vi "2d_Init.vi"(8 "error in (no error)":errorcluster, 11 "MagSpec_Bella in":refnum<class "MagSpec_Bella.lvclass">) -> (0 "error out":errorcluster, 3 "MagSpec_Bella out":refnum<class "MagSpec_Bella.lvclass">)   [LabVIEW 2020, in "MagSpec_Bella.lvclass"]
uses:
  MagSpec_Bella.lvclass
  MagSpec_Bella.lvclass/MagSpec_Bella.ctl
  2D.ctl
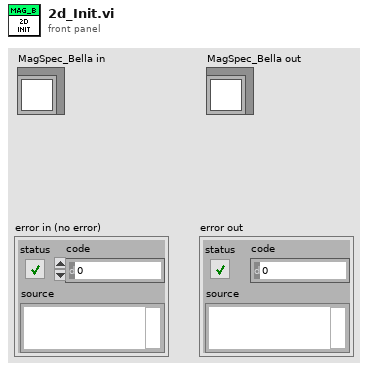
[diagram p1: front panel]
types:
  T1 = typedef "CameraSettings_File.ctl" = cluster{"FOV [mm]":dbl, "Left edge [mm]":dbl, "ROI Y offset":dbl, "ROI height":dbl, "ROI X offset":dbl, "ROI width":dbl, "Y center pixel":dbl, "Y Start":dbl, "Y End":dbl, "X Start":dbl, "X End":dbl, "rot [deg]":dbl}
  T2 = typedef "Calibration_Pixel_based.ctl" = cluster{"y1(pixel)":dbl[], "y2(pixel)":dbl[], "dp/B [MeV/C/B] (pixel)":dbl[], "energyDependence Input(pixel)":dbl[], "bending angle [deg](pixel)":dbl[], "total path(pixel)":dbl[], "pixel angle (y)(pixel)":dbl[], "energy dependence (pixel)":dbl[], "charge compensation (pixel)":dbl[], "Momentum [MeV/C](pixel)":dbl[], "angular compensation(pixel)":dbl[]}
  T3 = typedef "2D.ctl" = cluster{"dp":dbl[][], "chargeCompensation":dbl[][], "angle":dbl[][], "Momentum":dbl[][]}
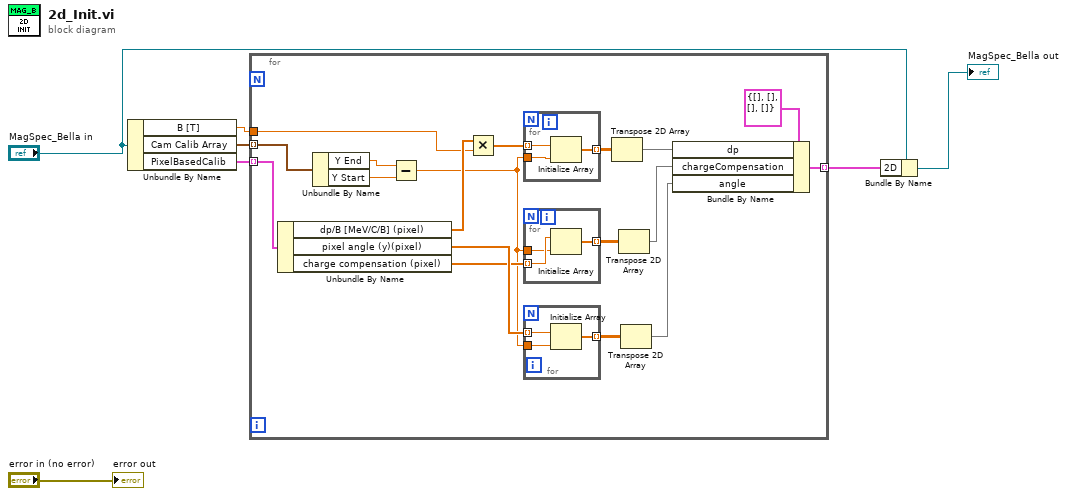
[diagram p0: block diagram]
diagram:
  n1 = Unbundle By Name("MagSpec_Bella in") -> ("B [T]"=w2:dbl, "Cam Calib Array"=w4:T1[], "PixelBasedCalib"=w5:T2[])
  n2 = for {
    tunnel: w4 -> [w15] mode=indexing
    tunnel: w2 -> [w14]
    tunnel: w5 -> [w13] mode=indexing
    tunnel: [w11] -> w1 mode=indexing
    n3 = Unbundle By Name(w13) -> ("dp/B [MeV/C/B] (pixel)"=w17:dbl[], "pixel angle (y)(pixel)"=w21:dbl[], "charge compensation (pixel)"=w16:dbl[])
    n4 = Unbundle By Name(w15) -> ("Y End"=w10:dbl, "Y Start"=w8:dbl)
    n5 = Subtract(x=w10, y=w8) -> (x-y=w9:dbl)
    n6 = Multiply(x=w17, y=w14) -> (x*y=w23:dbl[])
    n7 = for {
      tunnel: w23 -> [w31] mode=indexing
      tunnel: [w30] -> w24 mode=indexing
      tunnel: w9 -> [w29]
      n8 = Initialize Array(w31, w29) -> (w30:dbl[])
    }
    n9 = for {
      tunnel: w16 -> [w28] mode=indexing
      tunnel: [w27] -> w22 mode=indexing
      tunnel: w9 -> [w26]
      n10 = Initialize Array(w28, w26) -> (w27:dbl[])
    }
    n11 = for {
      tunnel: w21 -> [w34] mode=indexing
      tunnel: [w33] -> w25 mode=indexing
      tunnel: w9 -> [w32]
      n12 = Initialize Array(w34, w32) -> (w33:dbl[])
    }
    n13 = Transpose 2D Array(2D array=w24) -> (transposed array=w20:dbl[][])
    n14 = Transpose 2D Array(2D array=w22) -> (transposed array=w18:dbl[][])
    n15 = Transpose 2D Array(2D array=w25) -> (transposed array=w19:dbl[][])
    n16 = Bundle By Name(cluster=T3 {"dp"=[], "chargeCompensation"=[], "angle"=[], "Momentum"=[]} ("2D"), "dp"=w20, "chargeCompensation"=w18, "angle"=w19) -> (w11:T3)
  }
  n17 = Bundle By Name(cluster="MagSpec_Bella in", "2D"=w1) -> (→"MagSpec_Bella out":refnum<class "MagSpec_Bella.lvclass">)
  "error out" <- "error in (no error)"
